vi "Read Drive PID.vi"() -> (3 "Cluster":T1)   [LabVIEW 2017]
uses:
  <vilib>/Rock Robotics/Network Tables/NT Read Number.vi
  <vilib>/Rock Robotics/Network Tables/NT Read Numeric Array.vi
panel:
  in  "Max Speed":dbl=0.7
  in  "PID":dbl[](array[numeric])
  in  "Min Speed":dbl=0.35
  in  "Accel Distance":dbl=64.0
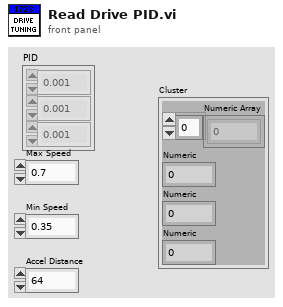
[diagram p1: front panel]
types:
  T1 = cluster{"Numeric Array":dbl[], "Numeric":dbl, "Numeric":dbl, "Numeric":dbl}
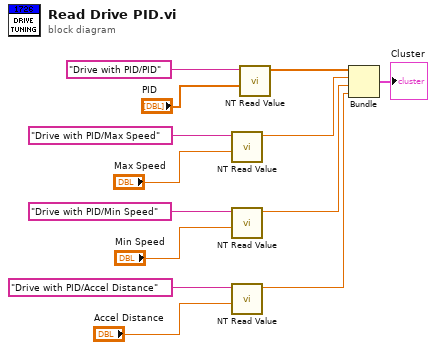
[diagram p0: block diagram]
diagram:
  n1 = call-poly <vilib>:"NT Read Value.vi"("Default Value"="Max Speed", "Name"="Drive with PID/Max Speed") -> ("Numeric"=w6:dbl)  [unwired: 8 in, 1 out]
  n2 = call-poly <vilib>:"NT Read Value.vi"("Default Value"="Min Speed", "Name"="Drive with PID/Min Speed") -> ("Numeric"=w7:dbl)  [unwired: 8 in, 1 out]
  n3 = call-poly <vilib>:"NT Read Value.vi"("Default Value"="Accel Distance", "Name"="Drive with PID/Accel Distance") -> ("Numeric"=w8:dbl)  [unwired: 8 in, 1 out]
  n4 = call-poly <vilib>:"NT Read Value.vi"("Default Value"="PID", "Name"="Drive with PID/PID") -> ("Numeric Array"=w5:dbl[])  [unwired: 8 in, 1 out]
  n5 = Bundle("Numeric Array"=w5, "Numeric"=w6, "Numeric"=w7, "Numeric"=w8) -> (→"Cluster":T1)  [unwired: 1 in]
